vi "All SubFunctions 5.vi"(8 "error":errorcluster, 9 "lines 1":tag="PXI1Slot8/port0/line2", 10 "lines":tag="PXI1Slot8/port0/line3", 11 "Path for Log":path) -> (0 "error IO":errorcluster, 1 "appended array 1":string[][](array[string]), 2 "appended array":string[][](array[string]))   [LabVIEW 2015]
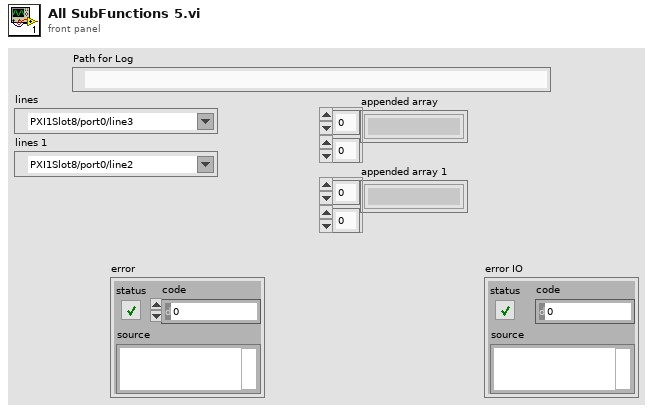
[diagram p1: front panel]
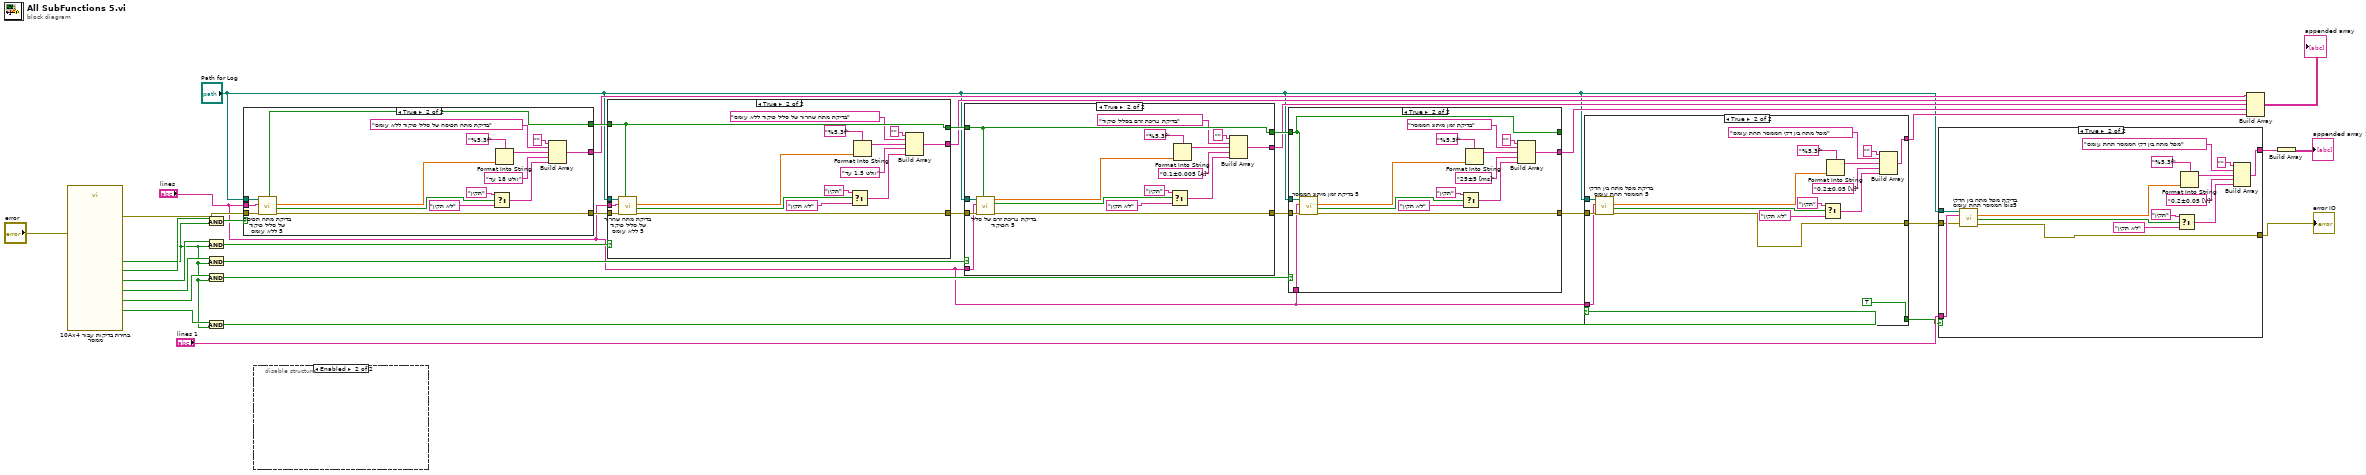
[diagram p0: block diagram]
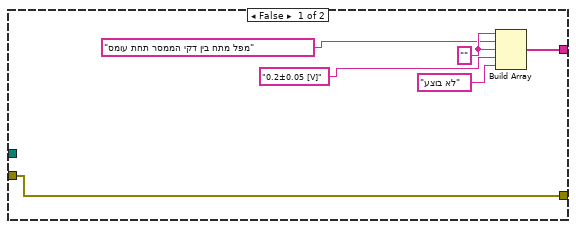
[diagram p2: hidden frame]
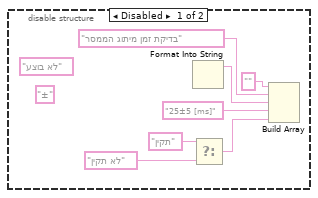
[diagram p3: hidden frame]
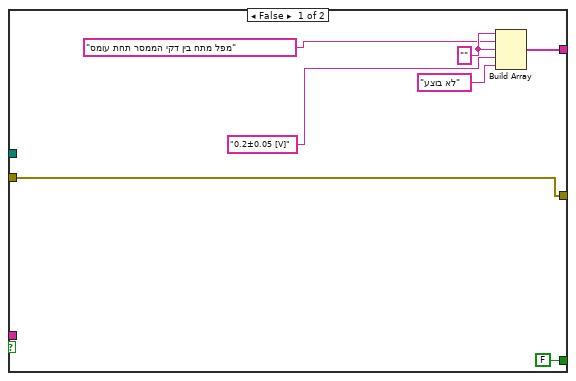
[diagram p4: hidden frame]
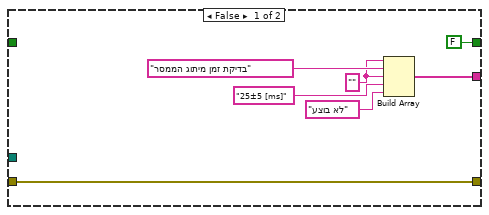
[diagram p5: hidden frame]
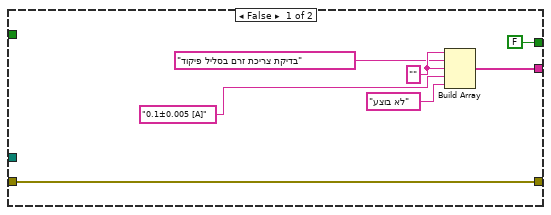
[diagram p6: hidden frame]
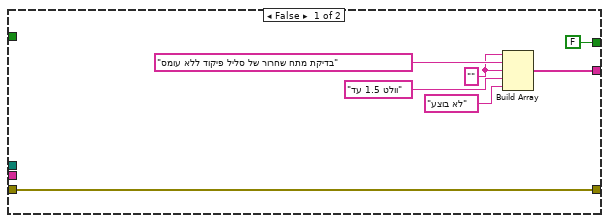
[diagram p7: hidden frame]
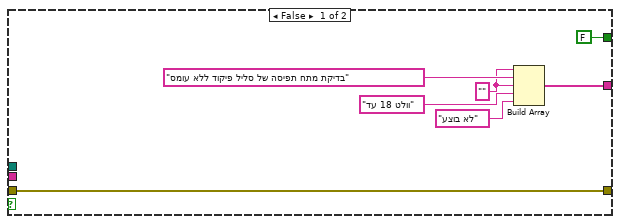
[diagram p8: hidden frame]
diagram:
  n1 = call "10Ax4 בחירת בדיקות עבור ממסר.vi"("error in (no error)"="error") -> ("בדיקת מפל מתח בין דקי הממסר תחת עומס"=w22:bool, "בדיקת זמן מיתוג הממסר"=w24:bool, "בדיקת צריכת זרם של סליל הפיקוד"=w26:bool, "בדיקת מתח שחרור של סליל פיקוד ללא עומס"=w28:bool, "בדיקת מתח תפיסה של סליל פיקוד ללא עומס"=w21:bool, "OK"=w20:bool, "error out"=w30:errorcluster)  [unwired: 11 in, 1 out]
  n2 = And(x=w21, y=w20) -> (x .and. y?=w29:bool)
  n3 = And(x=w28, y=w20) -> (x .and. y?=w27:bool)
  n4 = And(x=w26, y=w20) -> (x .and. y?=w25:bool)
  n5 = And(x=w24, y=w20) -> (x .and. y?=w23:bool)
  n6 = And(x=w22, y=w20) -> (x .and. y?=w7:bool)
  n7 = case shown="True" w29 {
    tunnel: [w41 w57] -> w32
    tunnel: w30 -> [w41 w56]
    tunnel: "Path for Log" -> [_ w55]
    tunnel: [FALSE ("resultUserPrompt") w54] -> w19
    tunnel: [w37 w44] -> w16
    tunnel: "lines" -> [_ w42]
    frame False {
      w36 = "" ("element")
      n8 = Build Array(w36, "בדיקת מתח תפיסה של סליל פיקוד ללא עומס" ("element"), w36, "עד 18 וולט" ("element"), "לא בוצע") -> (w37:string[])
    }
    frame True {
      n9 = call "בדיקת מתח תפיסה של סליל פיקוד ללא עומס 5.vi"("error"=w56, "lines"=w42, "Path for Log"=w55) -> ("error out"=w57:errorcluster, "מצב ממסר פתוח/סגור"=w51:bool, "מתח סגירת הממסר"=w50:dbl, "resultUserPrompt"=w54:bool)  [unwired: 4 in, 1 out]
      n10 = Select(t="תקין", s=w51, f="לא תקין") -> (s? t:f=w45:string)
      n11 = Format Into String(format string="%5.3f", w50) -> (resulting string=w46:string)  [unwired: 2 in, 1 out]
      n12 = Build Array("" ("element"), "בדיקת מתח תפיסה של סליל פיקוד ללא עומס" ("element"), w46, "עד 18 וולט" ("element"), w45) -> (w44:string[])
    }
  }
  n13 = disable-structure shown="Enabled" {
    frame Disabled {
      (unwired) "±"
      (unwired) "לא בוצע"
      n14 = Format Into String() -> (resulting string=w62:string)  [unwired: 4 in, 1 out]
      n15 = Select(t="תקין", f="לא תקין") -> (s? t:f=w64:string)  [unwired: 1 in]
      n16 = Build Array("" ("element"), "בדיקת זמן מיתוג הממסר" ("element"), w62, "25±5 [ms]" ("element"), w64) -> ()  [unwired: 1 out]
    }
    frame Enabled {
    }
  }
  n17 = case shown="True" w27 {
    tunnel: w32 -> [w71 w87]
    tunnel: [w71 w86] -> w31
    tunnel: "Path for Log" -> [_ w85]
    tunnel: w19 -> [_ w84]
    tunnel: [FALSE ("resultUserPrompt") w84] -> w18
    tunnel: [w65 w74] -> w15
    tunnel: "lines" -> [_ w72]
    frame False {
      w66 = "" ("element")
      n18 = Build Array(w66, "בדיקת מתח שחרור של סליל פיקוד ללא עומס" ("element"), w66, "עד 1.5 וולט" ("element"), "לא בוצע") -> (w65:string[])
    }
    frame True {
      n19 = call "בדיקת מתח שחרור של סליל פיקוד ללא עומס 5.vi"("resultUserPrompt"=w84, "error"=w87, "lines"=w72, "Path for Log"=w85) -> ("error out"=w86:errorcluster, "מצב ממסר פתוח/סגור"=w80:bool, "מתח פתיחת הממסר"=w81:dbl)  [unwired: 4 in, 1 out]
      n20 = Select(t="תקין", s=w80, f="לא תקין") -> (s? t:f=w75:string)
      n21 = Format Into String(format string="%5.3f", w81) -> (resulting string=w77:string)  [unwired: 2 in, 1 out]
      n22 = Build Array("" ("element"), "בדיקת מתח שחרור של סליל פיקוד ללא עומס" ("element"), w77, "עד 1.5 וולט" ("element"), w75) -> (w74:string[])
    }
  }
  n23 = case shown="True" w25 {
    tunnel: [w94 w110] -> w33
    tunnel: w31 -> [w94 w109]
    tunnel: "Path for Log" -> [_ w108]
    tunnel: w18 -> [_ w107]
    tunnel: [FALSE ("resultUserPrompt") w107] -> w17
    tunnel: [w89 w97] -> w14
    tunnel: "lines" -> [_ w95]
    frame False {
      w92 = "" ("element")
      n24 = Build Array(w92, "בדיקת צריכת זרם בסליל פיקוד" ("element"), w92, "0.1±0.005 [A]" ("element"), "לא בוצע") -> (w89:string[])
    }
    frame True {
      n25 = call "בדיקת צריכת זרם של סליל הפיקוד 5.vi"("resultUserPrompt"=w107, "error"=w109, "lines"=w95, "Path for Log"=w108) -> ("error out"=w110:errorcluster, "צריכת זרם בסליל בטווח כן/לא"=w100:bool, "צריכת זרם בסליל"=w101:dbl)  [unwired: 5 in]
      n26 = Select(t="תקין", s=w100, f="לא תקין") -> (s? t:f=w99:string)
      n27 = Format Into String(format string="%5.3f", w101) -> (resulting string=w98:string)  [unwired: 2 in, 1 out]
      n28 = Build Array("" ("element"), "בדיקת צריכת זרם בסליל פיקוד" ("element"), w98, "0.1±0.005 [A]" ("element"), w99) -> (w97:string[])
    }
  }
  n29 = case shown="True" w23 {
    tunnel: w33 -> [w117 w133]
    tunnel: [w117 w132] -> w12
    tunnel: "Path for Log" -> [_ w131]
    tunnel: w17 -> [_ w119]
    tunnel: [FALSE ("resultUserPrompt") w119] -> _
    tunnel: [w111 w121] -> w13
    tunnel: "lines" -> [_ w118]
    frame False {
      w113 = "" ("element")
      n30 = Build Array(w113, "בדיקת זמן מיתוג הממסר" ("element"), w113, "25±5 [ms]" ("element"), "לא בוצע") -> (w111:string[])
    }
    frame True {
      n31 = call "בדיקת זמן מיתוג הממסר 5.vi"("resultUserPrompt"=w119, "error"=w133, "lines"=w118, "Path for Log"=w131) -> ("error out"=w132:errorcluster, "בטוח כן/לא"=w123:bool, "בדיקת זמן מיתוג הממסר"=w122:dbl)  [unwired: 5 in]
      n32 = Select(t="תקין", s=w123, f="לא תקין") -> (s? t:f=w124:string)
      n33 = Format Into String(format string="%5.3f", w122) -> (resulting string=w126:string)  [unwired: 2 in, 1 out]
      n34 = Build Array("" ("element"), "בדיקת זמן מיתוג הממסר" ("element"), w126, "25±5 [ms]" ("element"), w124) -> (w121:string[])
    }
  }
  n35 = case shown="True" w7 {
    tunnel: [w140 w141] -> w6
    tunnel: w12 -> [w140 w156]
    tunnel: "Path for Log" -> [_ w155]
    tunnel: [w137 w145] -> w11
    tunnel: "lines" -> [_ w143]
    tunnel: [FALSE TRUE] -> w2
    frame False {
      w138 = "" ("element")
      n36 = Build Array(w138, "מפל מתח בין דקי הממסר תחת עומס" ("element"), w138, "0.2±0.05 [V]" ("element"), "לא בוצע") -> (w137:string[])
    }
    frame True {
      n37 = call "בדיקת מפל מתח בין הדקי הממסר תחת עומס 5.vi"("error"=w156, "lines"=w143, "Path for Log"=w155) -> ("error IO"=w141:errorcluster, "בטוח כן/לא"=w146:bool, "מפל מתח בין דקי הממסר תחת עומס"=w147:dbl)  [unwired: 5 in, 1 out]
      n38 = Select(t="תקין", s=w146, f="לא תקין") -> (s? t:f=w148:string)
      n39 = Format Into String(format string="%5.3f", w147) -> (resulting string=w150:string)  [unwired: 2 in, 1 out]
      n40 = Build Array("" ("element"), "מפל מתח בין דקי הממסר תחת עומס" ("element"), w150, "0.2±0.05 [V]" ("element"), w148) -> (w145:string[])
    }
  }
  n41 = case shown="True" w2 {
    tunnel: [w159 w163] -> w5
    tunnel: "Path for Log" -> [_ w177]
    tunnel: [w160 w167] -> w4
    tunnel: "lines 1" -> [_ w165]
    tunnel: w6 -> [w159 w164]
    frame False {
      w161 = "" ("element")
      n42 = Build Array(w161, "מפל מתח בין דקי הממסר תחת עומס" ("element"), w161, "0.2±0.05 [V]" ("element"), "לא בוצע") -> (w160:string[])
    }
    frame True {
      n43 = call "בדיקת מפל מתח בין הדקי הממסר תחת עומס bis5.vi"("error"=w164, "lines"=w165, "Path for Log"=w177) -> ("error IO"=w163:errorcluster, "בטוח כן/לא"=w168:bool, "מפל מתח בין דקי הממסר תחת עומס"=w169:dbl)  [unwired: 5 in, 1 out]
      n44 = Select(t="תקין", s=w168, f="לא תקין") -> (s? t:f=w170:string)
      n45 = Format Into String(format string="%5.3f", w169) -> (resulting string=w172:string)  [unwired: 2 in, 1 out]
      n46 = Build Array("" ("element"), "מפל מתח בין דקי הממסר תחת עומס" ("element"), w172, "0.2±0.05 [V]" ("element"), w170) -> (w167:string[])
    }
  }
  "error IO" <- w5
  n47 = Build Array(w16, w15, w14, w13, w11) -> (→"appended array":string[][])
  n48 = Build Array(w4) -> (→"appended array 1":string[][])
